vi "Robot Main.vi"() -> ()   [LabVIEW 2011]
doc: "This VI imlements the framework and scheduler for your robotics program. It should not be necessary to modify the framework. You are expected to add your code to the VIs called from Robot Main, the ones located in the Team Code within the project."
uses:
  Robot Global Data.vi
panel:
  out "Robot Main Timer":u32
  in  "Finish":bool
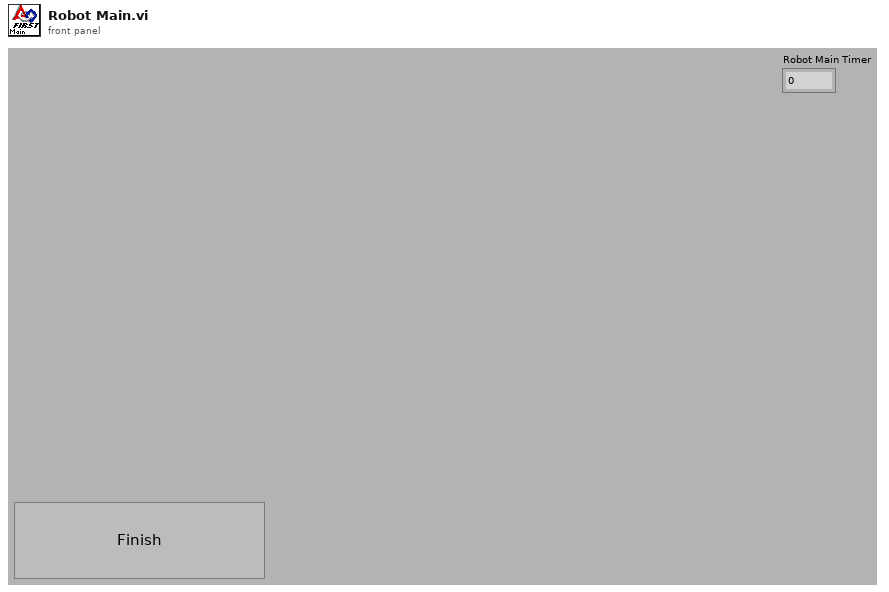
[diagram p1: front panel]
types:
  T1 = typedef "WPI_GyroDevRef.ctl" = cluster{"DevStatus":errorcluster, "Analog Module":T2, "Analog Channel":T3, "Offset":dbl, "Gain (VoltsPerDegree/Second)":dbl}
  T2 = typedef "FPGA_TypedefAnalogModule.ctl" = enum16{"Analog Module 1", "Analog Module 2"}
  T3 = typedef "FPGA_AIChannel.ctl" = enum8{"AI 1", "AI 2", "AI 3", "AI 4", "AI 5", "AI 6", "AI 7", "AI 8", "Invalid"}
  T4 = typedef "WPI_EncoderDevRef.ctl" = cluster{"DevStatus":errorcluster, "EncoderIndex":T5, "CounterIndex":T6, "DistancePerCount":dbl, "Decoding Type":T7}
  T5 = typedef "FPGA_EncoderIdx.ctl" = enum8{"Enc 0", "Enc 1", "Enc 2", "Enc 3", "Invalid"}
  T6 = typedef "FPGA_CounterCtrSystemIndex.ctl" = enum8{"Ctr 0", "Ctr 1", "Ctr 2", "Ctr 3", "Ctr 4", "Ctr 5", "Ctr 6", "Ctr 7", "Invalid"}
  T7 = typedef "WPI_EncoderType.ctl" = enum16{"1x", "2x", "4x"}
  T8 = typedef "WPI_DriverStationMatch Info.ctl" = cluster{"Autonomous Elapsed Seconds":dbl, "TeleOp Elapsed Seconds":dbl, "Disabled Elapsed Seconds":dbl, "Visited Autonomous":bool, "Visited TeleOp":bool, "Visited Disabled":bool, "Autonomous Settings":cluster{"Autonomous Style":enum16{"Iterative", "Independent"}, "VI Refnum":refnum<vi>}}
  T9 = typedef "WPI_DriverStationDerivedRobotMode.ctl" = enum16{"Init", "Execute", "Stop"}
  T10 = typedef "WPI_DriverStationRobotMode.ctl" = enum16{"Autonomous Disabled", "Autonomous Enabled", "Teleop Disabled", "Teleop Enabled", "Timeout", "Finish"}
  T11 = typedef "WPI_CameraDevRef.ctl" = cluster{"Camera Address":string, "CameraStatus":errorcluster, "Acquire Image Notifier":refnum<notifier>}
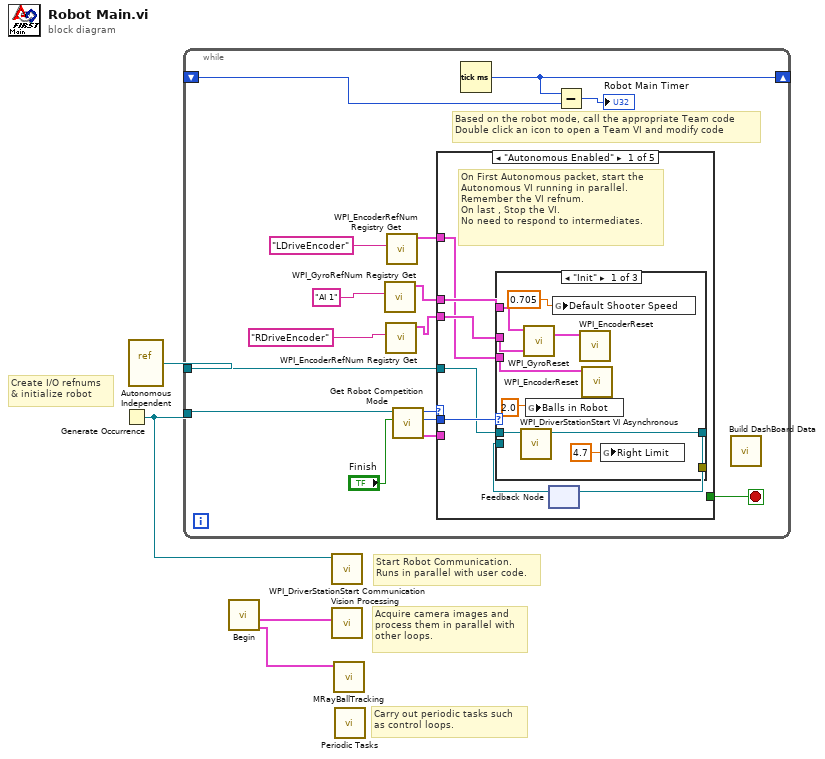
[diagram p0: block diagram]
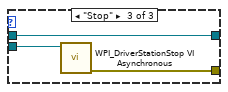
[diagram p3: hidden frame]
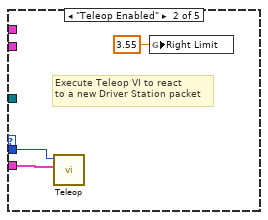
[diagram p4: hidden frame]
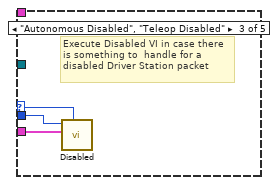
[diagram p5: hidden frame]
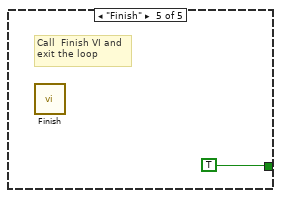
[diagram p7: hidden frame]
diagram:
  # "Acquire camera images and\nprocess them in parallel with\nother loops."
  # "Create I/O refnums\n& initialize robot"
  # "Carry out periodic tasks such\nas control loops."
  # "Start Robot Communication.\nRuns in parallel with user code."
  n1 = Generate Occurrence() -> (w4:refnum<k4>)
  n2 = vi-ref "Autonomous Independent.vi"() -> (w3:refnum<vi>)
  n3 = while {
    tunnel: w4 -> [w18]
    tunnel: w3 -> [w14]
    shift-right: [w13] -> _
    shift-left: _ -> [w12]
    stop <- w15 stop-if-true
    # "Based on the robot mode, call the appropriate Team code\nDouble click an icon to open a Team VI and modify code"
    n4 = call <vilib>:"WPI_GyroRefNum Registry Get.vi"("refnum name"="AI 1") -> ("GyroDevRef"=w10:T1)  [unwired: 9 in, 1 out]
    n5 = call <vilib>:"WPI_EncoderRefNum Registry Get.vi"("refnum name"="RDriveEncoder") -> ("EncoderDevRef"=w9:T4)  [unwired: 9 in, 1 out]
    n6 = call <vilib>:"WPI_EncoderRefNum Registry Get.vi"("refnum name"="LDriveEncoder") -> ("EncoderDevRef"=w8:T4)  [unwired: 9 in, 1 out]
    n7 = call "Get Robot Competition Mode.vi"("Finish"="Finish", "DS Occurrence"=w18) -> ("Match Info out"=w16:T8, "Call Context"=w20:T9, "Robot Mode"=w19:T10)  [unwired: 7 out]
    n8 = case shown="\"Autonomous Enabled\"" w19 {
      selector: w19 -> [_ _ w43 _ _]
      tunnel: w20 -> [w27 w42 w45 _ _]
      tunnel: w16 -> [_ w41 w44 _ _]
      tunnel: [_ _ _ _ TRUE] -> w15
      tunnel: w14 -> [w26 _ _ _ _]
      tunnel: w10 -> [w23 _ _ _ _]
      tunnel: w9 -> [w22 _ _ _ _]
      tunnel: w8 -> [w21 _ _ _ _]
      frame "Autonomous Enabled" {
        # "On First Autonomous packet, start the\nAutonomous VI running in parallel.\nRemember the VI refnum.\nOn last , Stop the VI.\nNo need to respond to intermediates."
        n9 = feedback #1() -> (w24:refnum<vi>)  [unwired: 1 out]
        n10 = case shown="\"Init\"" w27 {
          tunnel: w26 -> [w35 _ w38]
          tunnel: [w34 w36 w38] -> w25
          tunnel: w24 -> [_ w36 w39]
          tunnel: [_ _ w37] -> _
          tunnel: w23 -> [w33 _ _]
          tunnel: w22 -> [w32 _ _]
          tunnel: w21 -> [w31 _ _]
          frame "Init" {
            n11 = call <vilib>:"WPI_DriverStationStart VI Asynchronous.vi"("VI"=w35) -> ("VI out"=w34:refnum<vi>)  [unwired: 10 out]
            n12 = call <vilib>:"WPI_GyroReset.vi"("GyroDevRef"=w33) -> ()  [unwired: 9 in, 2 out]
            n13 = global write "Robot Global Data.vi" "Balls in Robot"(2.0 ("Right Limit")) -> ()
            n14 = global write "Robot Global Data.vi" "Default Shooter Speed"(0.705 ("Balls in Robot")) -> ()
            n15 = call <vilib>:"WPI_EncoderReset.vi"("EncoderDevRef"=w32) -> ()  [unwired: 9 in, 2 out]
            n16 = call <vilib>:"WPI_EncoderReset.vi"("EncoderDevRef"=w31) -> ()  [unwired: 9 in, 2 out]
            n17 = global write "Robot Global Data.vi" "Right Limit"(4.7 ("Right Limit")) -> ()
          }
          frame "Execute", Default {
            # "Nothing to do"
          }
          frame "Stop" {
            n18 = call <vilib>:"WPI_DriverStationStop VI Asynchronous.vi"("VI Refnum"=w39) -> ("error out"=w37:errorcluster)  [unwired: 10 out]
          }
        }
        n19 = feedback-in #1(w25) -> ()
      }
      frame "Teleop Enabled" {
        # "Execute Teleop VI to react\nto a new Driver Station packet"
        n20 = call "Teleop.vi"("Match Info"=w41, "Call Context"=w42) -> ()  [unwired: 1 in, 9 out]
        n21 = global write "Robot Global Data.vi" "Right Limit"(3.55 ("Right Limit")) -> ()
      }
      frame "Autonomous Disabled", "Teleop Disabled" {
        # "Execute Disabled VI in case there\nis something to  handle for a\ndisabled Driver Station packet"
        n22 = call "Disabled.vi"("Robot Mode"=w43, "Match Info"=w44, "Call Context"=w45) -> ()  [unwired: 1 in, 8 out]
      }
      frame "Timeout" {
        # "Driver Station packet didn't arrive.\nPossibly useful for diagnostics"
      }
      frame "Finish" {
        # "Call  Finish VI and\nexit the loop"
        n23 = call "Finish.vi"() -> ()  [unwired: 1 in, 7 out]
      }
    }
    n24 = Tick Count (ms)() -> (millisecond timer value=w13:u32)
    n25 = Subtract(x=w13, y=w12) -> (x-y=→"Robot Main Timer":u32)
    n26 = call "Build DashBoard Data.vi"() -> ()  [unwired: 1 in, 11 out]
  }
  n27 = call "Begin.vi"() -> ("CameraDevRef 2"=w1:T11, "CameraDevRef"=w2:T11)  [unwired: 1 in, 9 out]
  n28 = call <vilib>:"WPI_DriverStationStart Communication.vi"("occurrence"=w4) -> ()  [unwired: 11 out]
  n29 = call "Vision Processing.vi"("CameraDevRef"=w2) -> ()  [unwired: 2 in, 5 out]
  n30 = call "MRayBallTracking.vi"("CameraDevRef"=w1) -> ()  [unwired: 11 in]
  n31 = call "Periodic Tasks.vi"() -> ()  [unwired: 2 in, 10 out]
